vi "Data Collection with cDAQ for Training.vi"() -> ()   [LabVIEW 2024]
uses:
  <vilib>/Utility/error.llb/DialogType.ctl
  <vilib>/DAQmx/write.llb/DAQmx Write (Analog DBL 1Chan 1Samp).vi
  <vilib>/DAQmx/read.llb/DAQmx Read (Analog 2D DBL NChan NSamp).vi
  <vilib>/DAQmx/create/channels.llb/DAQmx Create Channel (AI-Voltage-Basic).vi
  <vilib>/DAQmx/configure/timing.llb/DAQmx Timing (Sample Clock).vi
  <vilib>/DAQmx/create/channels.llb/DAQmx Create Channel (AO-Voltage-Basic).vi
  <vilib>/DAQmx/miscellaneous.llb/DAQmx Fill In Error Info.vi
panel:
  out "Voltage":dbl
  in  "Fan speed channel":tag="cDAQ9188-18973A7Mod1/ao0"
  in  "to":dbl=5.0 format="%#_13g"
  in  "From":dbl=1.7 format="%#_13g"
  in  "Labels/Class":i64(slide) scale=0.0..1.0
  out "Waveform Graph":dbl[][](graph)=[[2.465981210666, 2.474281700632, 2.474497052165, 2.485680690417, 2.507517823912, 2.502643436522, 2.4864865809979997, 2.481108893283, 2.479818614268, 2.4730475472289997, 2.4604876113609997, 2.4396686696749996, 2.4241749504579997, 2.4281263155549997, 2.444756578415, 2.453837946461, 2.4663466372049996, 2.4774448669169997, 2.4748167241289996, 2.484621624521, 2.506576499789, 2.504133815545, 2.485150547408, 2.483149547328, 2.4809856609609997, 2.472076940178, 2.457618494478, 2.435155438397, 2.4250949224459997, 2.4324162645069998, 2.4408338861849996, 2.45345299797, 2.467477690299, 2.475509143364, 2.4749503274879996, 2.489877910097, 2.5070474668809997, 2.4995546976789997, 2.4889463469499997, 2.4833526976409996, 2.480550687468, 2.4680060031249997, 2.4576441170399996, 2.4361358064239997, 2.4244787608359997, 2.434380660927, 2.4408064334399997, 2.4532108037529996, 2.4677650290299997, 2.4768512775639997, 2.477951217547, 2.4870813904729996, 2.5042344756099997, 2.499357647976, 2.486270009343, 2.4847143537929997, 2.4789541578309997, 2.4667968622229997, 2.456221454788, 2.434156158479, 2.4231122241959997, 2.4336589587639996, 2.4417257953669997, 2.451367809472, 2.467566149144, 2.4797142938369996, 2.479826545061, 2.487126534987, 2.5040691490789997, 2.5002196641689998, 2.4886913414519998, 2.4841738397469997, 2.4788931517309996, 2.4651545780109996, 2.4557327959269997, 2.4338694298089996, 2.4233050034719996, 2.4352609789499997, 2.4439763103959997, 2.453197992472, 2.468630095528, 2.4780158840129998, 2.476577970236, 2.488984780793, 2.5052929314449996, 2.4992783400459997, 2.4873004023719996, 2.485744136761, 2.4785204044599998, 2.467098232357, 2.456855308167, 2.4335381666859996, 2.424061479112, 2.435603833232, 2.4427214149189997, 2.45535028768, 2.4709849309879997, 2.4791591383269997, 2.4783007825, 2.489077510065, 2.508760518169, 2.5018588980759997, 2.4863566380049997, 2.483073899764, 2.478242826705, 2.467089081442, 2.4589661192269996, 2.4329128541609997, 2.4242872016819996, 2.432615754454, 2.4475360163309996, 2.4560231849629997, 2.468813113828, 2.474465328993, 2.4772539178239996, 2.4906654988479997, 2.5083066327849997, 2.4981399662199997, 2.4845581781769996, 2.483920664432, 2.4776370361319997, 2.4677790604329997, 2.4557547581229997, 2.431507883678, 2.424400062967, 2.434973640219, 2.4427000627839996, 2.456904723108, 2.469652557764, 2.475894091855, 2.4742493673989996, 2.4918355958459997, 2.5103783999409996, 2.497681810409, 2.4837321555829996, 2.4847186242199997, 2.478000632488, 2.469579960505, 2.4536793306009996, 2.432682251103, 2.4226211250909997, 2.433942027068, 2.445550267776, 2.457020634698, 2.471956758161, 2.477662048633, 2.4740425567199997, 2.4942154438069997, 2.5074232644569996, 2.496548927132, 2.4838346458309997, 2.4816341558039996, 2.4795794703559997, 2.46584333688, 2.452324995181, 2.429816184525, 2.426056378582, 2.4354256954199998, 2.443791461913, 2.454458988559, 2.4712210245949997, 2.4793061630279998, 2.4790212645409997, 2.4921430665899997, 2.5086006821869997, 2.4960511173559996, 2.4845002223819996, 2.483541816551, 2.4789315855739997, 2.464736686226, 2.4503789005909997, 2.4311754004329997, 2.425056488603, 2.437829945821, 2.443725575325, 2.457002942929, 2.4724765301329996, 2.4779597584009996, 2.478148877311, 2.49261891417, 2.5054765598059996, 2.497401182349, 2.4842189842609996, 2.4848839507509997, 2.4760661290569996, 2.4645158441439996, 2.4507058932869996, 2.4308014330399996, 2.4266267856169996, 2.437742707098, 2.443214954268, 2.45586883953, 2.4683092034419998, 2.478598492268, 2.481068629257, 2.491521414431, 2.5037208042479997, 2.4969875609909997, 2.487239396272, 2.48402925529, 2.4761112735709996, 2.465160678621, 2.4506473274309997, 2.4308050934059997, 2.4266450874469996, 2.4386449873169997, 2.4445393966989997, 2.45658871151, 2.4706890514029998, 2.478715013919, 2.478946837099, 2.49491884414, 2.5046407762359997, 2.4953593081819996, 2.483546086978, 2.483752897657, 2.4749539878539997, 2.46359221179, 2.4507284655439996, 2.430625735472, 2.427852398166, 2.434272070069, 2.44754150688, 2.4583853411549996, 2.473045717046, 2.4776693693649996, 2.478772969714, 2.496637996038, 2.5060908912329998, 2.4938616084269998, 2.48377913028, 2.4823338957709997, 2.4748368561419998, 2.466200222565, 2.4502910518069996, 2.428717464664, 2.426235736516, 2.4379769705219996, 2.4469826910039996, 2.4601752601289997, 2.470236996202, 2.4765566181009997, 2.4807483472319998, 2.496722184456, 2.5061555576989996, 2.495196421895, 2.48317516989, 2.483416143985, 2.4752565781099998, 2.463057798354, 2.4485481075299997, 2.429633776286, 2.4261271456579996, 2.4353829911499996, 2.4495126139709997, 2.46211586417, 2.470737246222, 2.475550627512, 2.481315093901, 2.4988982720429997, 2.507872269353, 2.491820344321, 2.4798064130479998, 2.483708363204, 2.475362118663, 2.464994742029, 2.4480521279369998, 2.4270227152059998, 2.428927935709, 2.439406343445, 2.448382170938, 2.4646805606139996, 2.4747172841859997, 2.475652507699, 2.4834899613659998, 2.499663898598, 2.5081907211949996, 2.491012013496, 2.4814590682969997, 2.48309586196, 2.4742981722789996, 2.4629791004849997, 2.4445698997489997, 2.4246532382819996, 2.4297387067779996, 2.4400932721309996, 2.4449646092159996, 2.4611312257159996, 2.474456788139, 2.475733645812, 2.4817274951369996, 2.4986127634949997, 2.507098101944, 2.492570719351, 2.4814895713469998, 2.4824992223019997, 2.472269109393, 2.461204433036, 2.4447315659139996, 2.427204513384, 2.429142677181, 2.4390390867229996, 2.44671182392, 2.4610952321169997, 2.4741017326369996, 2.480792881685, 2.483380760447, 2.499397912002, 2.5042222743899996, 2.4930551077849996, 2.4840805004139996, 2.4807587182689996, 2.471925034989, 2.461727255313, 2.44428378114, 2.42606125907, 2.4318806309489998, 2.440888791675, 2.449099602674, 2.46049920252, 2.4750735598099998, 2.4786106934879997, 2.4795263950489996, 2.4998713193379998, 2.5055869808469997, 2.4917916714539996, 2.483319144286, 2.480479920392, 2.4703992724279997, 2.4611129238859997, 2.4424456673469996, 2.4241121141749997, 2.4287650494219997, 2.440331195921, 2.4480094236669996, 2.462365379119, 2.4748832207779996, 2.477759658393, 2.4827768000569996, 2.500815693766, 2.5054844905989997, 2.4894191442249998, 2.48437699006, 2.481886721058, 2.470352297731, 2.4588093335499996, 2.4427134841259996, 2.4278408070069997, 2.430356698571, 2.4400218949939996, 2.4497639591029996, 2.464232165779, 2.4733873512059996, 2.477478420272, 2.482773139691, 2.502601952374, 2.5053551576669997, 2.4892855408659997, 2.4817665390409998, 2.482322304612, 2.471433325823, 2.4620158141659996, 2.443493142084, 2.4253236953209996, 2.4291707399869997, 2.4410565584499997, 2.4517765503419997, 2.4664625487949996, 2.472447857266, 2.4759447269179997, 2.485203622715, 2.5041283249959996, 2.503659798148, 2.4875938417129997, 2.481823274714, 2.480286531055, 2.470566429142, 2.4628546480409996, 2.442500572837, 2.4263278557269996, 2.428887061622, 2.44137989078, 2.452664189097, 2.465316244176, 2.4743335558169997, 2.4743915116119997, 2.485506823032, 2.5053557677279996, 2.5047023923969998, 2.4858386962159997, 2.481926375023, 2.482185650948, 2.4720598584699998, 2.4601795305559997, 2.4386004528639997, 2.4239931522799996, 2.429757618669, 2.4413255953509996, 2.4537513177989996, 2.466531485688, 2.476076500094, 2.4776736397919996, 2.48664031637, 2.50522277443, 2.5027788700639997, 2.4871570380369996, 2.4821996823509997, 2.4798393563419996, 2.472058028287, 2.457882650891, 2.4385119940189997, 2.42601245419, 2.429107293643, 2.441180400833, 2.452409183599, 2.465429105461, 2.4777352559529997, 2.4754633887889996, 2.486684850823, 2.504718864044, 2.502132815465, 2.488896321948, 2.4816829606839996, 2.481207723165, 2.469508583368, 2.4570676093949997, 2.43660311315, 2.423556348604, 2.432535836463, 2.442326095391, 2.4515770603949996, 2.4662209646389996, 2.4764596184019996, 2.480059588363, 2.4882557578979996, 2.503687250893, 2.499909753181, 2.4872058429169996, 2.4831147738509998, 2.4796331557239997, 2.467799802507, 2.4568858112169996, 2.4343336862299996, 2.423824165383, 2.433771820049, 2.442518264606, 2.450650377736, 2.4677217146989996, 2.478305662988, 2.477643136742, 2.486916674003, 2.504412003361, 2.500820574254, 2.488538216141, 2.485301232475, 2.4790651889329998, 2.4681536378869997, 2.4559505877039998, 2.4322198248649998, 2.4247636593229998, 2.433116614535, 2.4434675195219997, 2.452935056181, 2.4686593784559996, 2.4777126836959997, 2.4775443068599996, 2.486747687106, 2.505879810127, 2.5015197041599997, 2.485908853231, 2.4832544778199996, 2.4796508474929997, 2.4662880713489996, 2.455176420295, 2.4360882216659996, 2.421810354022, 2.432079510835, 2.4446742201799996, 2.454216794342, 2.4703199644979996, 2.4757135137989996, 2.4750345159059997, 2.4932832705989996, 2.5072487870109996, 2.4989269449099996, 2.4853445468059996, 2.480380480449, 2.478009783403, 2.4673410366349997, 2.4573305456859997, 2.432709093787, 2.421890882074, 2.4346179746559997, 2.4450341561699998, 2.4570859112249996, 2.4711850309959997, 2.477607753204, 2.4748606485209996, 2.4954386161119997, 2.5096945215599997], [2.5011656271239997, 2.482636647164, 2.478799677952, 2.474818113144, 2.46122917766, 2.4633871296559997, 2.465378522168, 2.4833883002199997, 2.516363417404, 2.5254540266039998, 2.5478205858839997, 2.560706676952, 2.560751214836, 2.568139012608, 2.5376104285039998, 2.513711277928, 2.500819695888, 2.482330983056, 2.4785165878399997, 2.47191216874, 2.461731296544, 2.4622328053199998, 2.466136886412, 2.485111245212, 2.5189453944599998, 2.5271891737559997, 2.5507979129239997, 2.56017039202, 2.5591856777079998, 2.564380747328, 2.5390057455, 2.5109810446279996, 2.497606257052, 2.4795391288479998, 2.4804713738719997, 2.473206817916, 2.461040654288, 2.46144271546, 2.462791664248, 2.486275331276, 2.5223418656959997, 2.529992620016, 2.550364736244, 2.557160119148, 2.559825681, 2.569013297372, 2.542601722052, 2.511970639804, 2.494566088888, 2.479243836576, 2.4808234061879997, 2.4750859505559997, 2.460962560464, 2.461443935676, 2.4615976828919996, 2.4897846724919996, 2.524060539932, 2.5302336126759997, 2.5499321696719996, 2.553287763672, 2.559644478924, 2.570312217304, 2.5388587094719997, 2.510466723584, 2.493937677648, 2.4773036931359997, 2.4816598642559997, 2.473870005312, 2.460740481152, 2.4612932389999997, 2.4609729323, 2.490006141696, 2.5255077161079997, 2.533063903688, 2.5494123576559997, 2.55170514352, 2.5603583052839998, 2.570497690136, 2.5402515860359998, 2.5097278827959997, 2.495518467476, 2.479207840204, 2.4825140154559997, 2.47400178864, 2.45944156122, 2.461005268024, 2.462209011108, 2.49071874784, 2.525763961468, 2.5313995290639997, 2.5502732200439997, 2.554422564552, 2.5615730303119997, 2.566006685148, 2.53672089104, 2.506393642576, 2.493772948488, 2.4759602353199996, 2.481636680152, 2.4702923319999996, 2.459278052276, 2.458411088808, 2.464710453908, 2.4932085985879997, 2.5239446194119997, 2.530483146848, 2.5502317327, 2.555534791436, 2.561749351524, 2.5649835340319997, 2.528884663888, 2.508403948436, 2.49704861834, 2.47917855502, 2.48039266994, 2.46905991384, 2.4591609115399997, 2.462393263724, 2.467432755804, 2.494243341756, 2.52212710768, 2.529295266572, 2.557805003304, 2.559646309248, 2.562161784532, 2.560347933448, 2.531283608544, 2.510603387776, 2.497996116064, 2.4790974106559998, 2.4808075433799996, 2.4682728745199998, 2.46139085628, 2.462953952976, 2.46628697298, 2.4964391204479996, 2.5233955222119997, 2.527466162788, 2.5545958352239997, 2.557166830336, 2.5638401916399998, 2.560453482132, 2.5288236530879997, 2.506850613468, 2.494876023752, 2.4792542084119997, 2.480353623028, 2.468618805756, 2.463612869616, 2.4643309667319997, 2.468044694128, 2.495868669468, 2.522251569712, 2.5320877308879997, 2.5563517260479998, 2.5563852819879997, 2.5626315676919997, 2.5623978963279996, 2.529920627272, 2.5077438115799997, 2.493330620188, 2.4783530788959998, 2.482709860124, 2.4695998594199997, 2.45898703076, 2.462648288868, 2.4664449909519996, 2.4978496901439997, 2.5252722144199997, 2.532113355424, 2.552494623272, 2.5556073942879998, 2.5634003037719997, 2.5604272474879997, 2.5285789997799997, 2.505708491292, 2.490795621448, 2.478042533924, 2.483970343252, 2.4704314366239997, 2.46164100056, 2.4617569210799997, 2.468061167044, 2.5001266132, 2.5287022415959997, 2.532017568468, 2.5515581074919997, 2.5515446851159997, 2.5640213937159997, 2.5646717688439997, 2.528885273996, 2.504984293096, 2.4928388731399997, 2.480266377584, 2.480723958584, 2.469280162828, 2.4619613072599997, 2.4618112206919998, 2.4669965285839996, 2.502049673616, 2.52868576868, 2.534586733256, 2.5507106674799997, 2.553643456636, 2.563087318368, 2.560810395312, 2.52708728572, 2.503075265164, 2.490449080104, 2.480643424328, 2.4821284271999997, 2.464803190324, 2.461112036924, 2.459198128128, 2.4717718439, 2.502576806928, 2.525541882156, 2.532741766664, 2.5519595585559998, 2.5547550734119997, 2.56291892856, 2.557506660492, 2.52590977728, 2.5065644728159997, 2.4921457904519997, 2.479981457148, 2.480347521948, 2.464794038704, 2.4609973366199998, 2.463379198252, 2.47031673632, 2.50316495104, 2.525372272132, 2.533747834756, 2.554426835308, 2.556368198964, 2.5616102469, 2.551886345596, 2.523813446192, 2.505316191848, 2.493494129132, 2.4788283530279998, 2.479907023972, 2.466773839164, 2.4634969490959997, 2.463043638852, 2.473727850148, 2.5048714231159996, 2.5243784062, 2.536736753848, 2.558921500944, 2.559442533176, 2.561827445348, 2.550979115, 2.519832491492, 2.508851767708, 2.4916436715679997, 2.477620339188, 2.479255428628, 2.4628063068399997, 2.462853895264, 2.4654590564239998, 2.47243686162, 2.504812852748, 2.522625565916, 2.535795357204, 2.55890441792, 2.558579230356, 2.5619342142479997, 2.548106116428, 2.518136391252, 2.5075351546439997, 2.489095250452, 2.47797664226, 2.4777814076999998, 2.4656579516319996, 2.463588465296, 2.4641515949799997, 2.4734472004679997, 2.5085820999719997, 2.524782907804, 2.5366751329399997, 2.557356573924, 2.557561570212, 2.563769419112, 2.5514013097359998, 2.5202339425559996, 2.50410451736, 2.4895540516679997, 2.479930818184, 2.4784671690919997, 2.464676897968, 2.463861183572, 2.463516472552, 2.474715615, 2.5108242468719997, 2.529236696204, 2.539082009, 2.5530418901479996, 2.555495744524, 2.567179922832, 2.5539857272239996, 2.517894788484, 2.5006208006799997, 2.48387638662, 2.478982100244, 2.478860078644, 2.4652009807399997, 2.462305408172, 2.4635213534159996, 2.477777747052, 2.512162213716, 2.528970689116, 2.5425602347079996, 2.552467168412, 2.554394499584, 2.568161586604, 2.55111943984, 2.5171650993159997, 2.500254125772, 2.4840899244199997, 2.480750803336, 2.479746565568, 2.46105224634, 2.460531214108, 2.4623737402679997, 2.477677079232, 2.51508341082, 2.52740759242, 2.54026866906, 2.55313279624, 2.55555187446, 2.5688595501559996, 2.5512018044199998, 2.518547604044, 2.5006586273759996, 2.4869104537039997, 2.4820320301359997, 2.4770974766319998, 2.4628917219599997, 2.461264563924, 2.463215689308, 2.47819628114, 2.517414633488, 2.526313058668, 2.5408342391759997, 2.556257769416, 2.5553383366599998, 2.5631428381959998, 2.5452642333639997, 2.5147234470999997, 2.503463293852, 2.4864821578879996, 2.482059484996, 2.47957512522, 2.46182098242, 2.459864366064, 2.464719605528, 2.479910074512, 2.515887533164, 2.52603484942, 2.54150108722, 2.556162592568, 2.557795851684, 2.564106198728, 2.541105127128, 2.515371991904, 2.503298564692, 2.4869940385, 2.479204179556, 2.47672592086, 2.46182098242, 2.4618557585759997, 2.467289380424, 2.4844889350519996, 2.51603822984, 2.5245120198519997, 2.5450159194079998, 2.559720742424, 2.5563328127, 2.560953160584, 2.5400716041759996, 2.514950407276, 2.504675578448, 2.4873588830839997, 2.479708738872, 2.472087879844, 2.4628648772079997, 2.465801327012, 2.466684763396, 2.481143712888, 2.5169045831999997, 2.5271891737559997, 2.54533256546, 2.5597164716679996, 2.561126431256, 2.560276550812, 2.5369801869399997, 2.512278134236, 2.502883691252, 2.482801986432, 2.478355519328, 2.4737681172759998, 2.4614927443159997, 2.465129598104, 2.4656384281759998, 2.4831936757679998, 2.517758124292, 2.528006108368, 2.546343514416, 2.556750126572, 2.5592595007759997, 2.5641336535879997, 2.540121633032, 2.5123672100039998, 2.499387162304, 2.482869098312, 2.479335962884, 2.47252837782, 2.463588465296, 2.464414551528, 2.462352996596, 2.4846304801079997, 2.5214901549279998, 2.5287852162839997, 2.546359987332, 2.5542663769039997, 2.56056086114, 2.566837042136, 2.537738551184, 2.510544817408, 2.49582840234, 2.4810680594959997, 2.480802052408, 2.472813298256, 2.462027809032, 2.462292595904, 2.4634341079719997, 2.4877511825279996, 2.523415045668, 2.53075098426, 2.546615622584, 2.5513043025639996, 2.55926438164, 2.569569715868, 2.541297921256, 2.509004294708, 2.494621608716, 2.47979171356, 2.480866723856, 2.475826621668, 2.460120001316, 2.4591340667879997, 2.463070483604, 2.4892557088559997, 2.523143547608, 2.5312134461239997, 2.550007823064, 2.552758189928, 2.560468734832, 2.56828482842, 2.538494474996, 2.507922573224, 2.494029803956, 2.4807251787999998, 2.48229925744, 2.4726424680159997, 2.459263409684, 2.4616117153759998, 2.463187014232, 2.4906089284, 2.526255708516, 2.531257984008, 2.550386700132, 2.556895332276, 2.561208185728, 2.5664746379839998, 2.5355073862279998, 2.508036053312, 2.495424510844, 2.480665998324, 2.480650135516, 2.470544306604, 2.459323810376, 2.462585447744, 2.464994154128, 2.4919359133, 2.525396676452, 2.5304489807999997, 2.5527215834479997, 2.5570533502479997, 2.564117180672, 2.5615083588639997, 2.531470301592, 2.50897622974, 2.495815590072, 2.478541602268, 2.478881432424, 2.46706791122, 2.461740448164]]
  in  "Stop":bool
  in  "Number of Samples":i32=500
  in  "Sample Rate":dbl=1000.0
  in  "Sample Clock Source":tag="OnboardClock"
  in  "Terminal Configuration":i32(ring)=-1 items=["default"=-1, "RSE"=10083, "NRSE"=10078, "Differential"=10106, "Pseudodifferential"=12529]
  in  "Max Voltage":dbl=5.0
  in  "Min Voltage":dbl=-5.0
  in  "Sensor channels":tag="cDAQ9188-18973A7Mod2/ai0:1"
  # "Fan Fault Detection: Data collection and labeling"
  # "Fault"
  # "Normal"
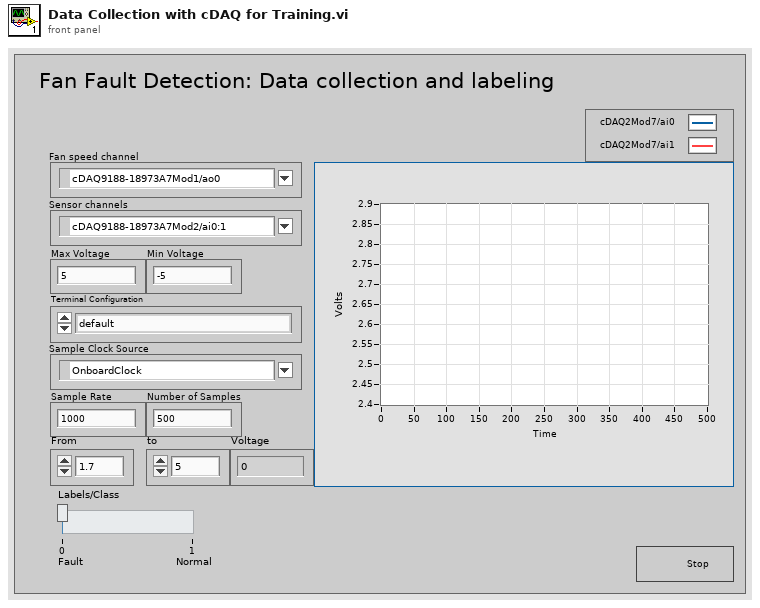
[diagram p1: front panel]
types:
  T1 = typedef "DialogType.ctl" = u16
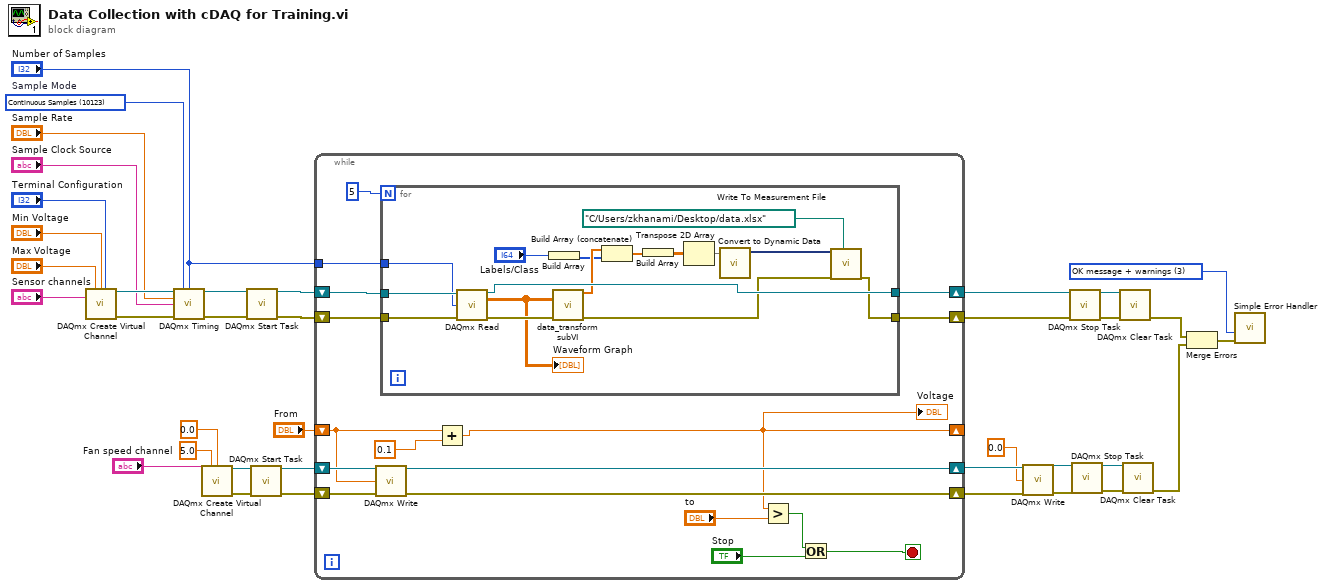
[diagram p0: block diagram]
diagram:
  w25 = T1 3 items=["no dialog", "OK message", "continue or stop message", "OK message + warnings", "continue/stop + warnings"] ("type of dialog (OK msg:1)")
  w37 = 10123 items=["Finite Samples"=10178, "Continuous Samples"=10123, "Hardware Timed Single Point"=12522]  # Sample Mode
  n1 = call-poly <vilib>:"DAQmx Create Virtual Channel.vi"("maximum value"="Max Voltage", "minimum value"="Min Voltage", "input terminal configuration"="Terminal Configuration", "physical channels"="Sensor channels") -> ("task out"=w35:refnum<k21>, "error out"=w36:errorcluster)  [unwired: 10 in]
  n2 = call-poly <vilib>:"DAQmx Timing.vi"("task/channels in"=w35, "sample mode"=w37, "samples per channel"="Number of Samples", "rate"="Sample Rate", "source"="Sample Clock Source", "error in"=w36) -> ("task out"=w24:refnum<k21>, "error out"=w23:errorcluster)  [unwired: 8 in]
  n3 = call-poly <vilib>:"DAQmx Create Virtual Channel.vi"("maximum value"=5.0, "minimum value"=0.0, "physical channels"="Fan speed channel") -> ("task out"=w14:refnum<k21>, "error out"=w15:errorcluster)  [unwired: 11 in]
  n4 = call <vilib>:"DAQmx Start Task.vi"("task/channels in"=w24, "error in"=w23) -> ("task out"=w22:refnum<k21>, "error out"=w19:errorcluster)  [unwired: 12 in]
  n5 = call <vilib>:"DAQmx Start Task.vi"("task/channels in"=w14, "error in"=w15) -> ("task out"=w13:refnum<k21>, "error out"=w16:errorcluster)  [unwired: 12 in]
  n6 = while {
    tunnel: "Number of Samples" -> [w54]
    shift-right: [w52] -> w21
    shift-left: w22 -> [w53]
    shift-right: [w51] -> w20
    shift-left: w19 -> [w50]
    shift-right: [w45] -> w3
    shift-left: w16 -> [w49]
    shift-right: [w44] -> w4
    shift-left: w13 -> [w48]
    shift-right: [w43] -> _
    shift-left: "From" -> [w47]
    stop <- w39 stop-if-true
    n7 = call-poly <vilib>:"DAQmx Write.vi"("task/channels in"=w48, "data"=w47, "error in"=w49) -> ("task out"=w44:refnum<k21>, "error out"=w45:errorcluster)  [unwired: 10 in, 1 out]
    n8 = for {
      N: 5 -> [_]
      tunnel: w53 -> [w70]
      tunnel: w54 -> [w69]
      tunnel: [w67] -> w52
      tunnel: [w59] -> w51
      tunnel: w50 -> [w65]
      n9 = call-poly <vilib>:"DAQmx Read.vi"("task/channels in"=w70, "number of samples per channel"=w69, "error in"=w65) -> ("task out"=w67:refnum<k21>, "data"=w56:dbl[][], "error out"=w68:errorcluster)  [unwired: 10 in]
      "Waveform Graph" <- w56
      n10 = Build Array("Labels/Class") -> (w62:i64[])
      n11 = call "data_transform subVI.vi"("data"=w56, "error in (no error)"=w68) -> ("Data"=w66:dbl[], "error out"=w60:errorcluster)  [unwired: 12 in]
      n12 = Build Array (concatenate)(w66, w62) -> (w63:dbl[])
      n13 = Build Array(w63) -> (w55:dbl[][])
      n14 = Transpose 2D Array(2D array=w55) -> (transposed array=w64:dbl[][])
      n15 = call "Convert to Dynamic Data"("2D Array"=w64) -> ("Dynamic Data Type"=w58:dynamicdata)  [unwired: 3 in]
      n16 = call "Write To Measurement File"("Signals"=w58, "error in (no error)"=w60, "Filename"=path "C:/Users/zkhanami/Desktop/data.xlsx") -> ("error out"=w59:errorcluster)  [unwired: 14 in, 2 out]
    }
    n17 = Add(x=w47, y=0.1) -> (x+y=w43:dbl)
    "Voltage" <- w43
    n18 = Greater?(x=w43, y="to") -> (0:w40:bool)
    n19 = Or(x=w40, y="Stop") -> (x .or. y?=w39:bool)
  }
  n20 = call-poly <vilib>:"DAQmx Write.vi"("task/channels in"=w4, "data"=0.0, "error in"=w3) -> ("task out"=w5:refnum<k21>, "error out"=w6:errorcluster)  [unwired: 10 in, 1 out]
  n21 = call <vilib>:"DAQmx Stop Task.vi"("task/channels in"=w21, "error in"=w20) -> ("task out"=w26:refnum<k21>, "error out"=w27:errorcluster)  [unwired: 12 in]
  n22 = call <vilib>:"DAQmx Stop Task.vi"("task/channels in"=w5, "error in"=w6) -> ("task out"=w10:refnum<k21>, "error out"=w11:errorcluster)  [unwired: 12 in]
  n23 = call <vilib>:"DAQmx Clear Task.vi"("task in"=w26, "error in"=w27) -> ("error out"=w8:errorcluster)  [unwired: 13 in]
  n24 = call <vilib>:"DAQmx Clear Task.vi"("task in"=w10, "error in"=w11) -> ("error out"=w9:errorcluster)  [unwired: 13 in]
  n25 = Merge Errors(w8, w9) -> (w7:errorcluster)
  n26 = call <vilib>:"Simple Error Handler.vi"("type of dialog (OK msg:1)"=w25, "error in (no error)"=w7) -> ()  [unwired: 3 in, 5 out]
